vi "Geometrical Analysis with Linear Programming.vi"() -> ()   [LabVIEW 2023]
doc: "Determines the solution of a linear programming problem and displays the solution."
uses:
  <vilib>/gmath/NI_Gmath.lvlib
panel:
  in  "Subject to constraints":string[](array[string])=["-x1 -x2<=-.6", "-x1 -1.5*x2<=-.65", "-x1 -2*x2<=-.8", "-x1 -4*x2<=-1.2", "0.1*x1 +0.2*x2>=.01"]
  out "Solution (x1,x2)":dbl[](array[numeric]) format="%#.6g"
  in  "Optimization Problem":u16(ring) items=["Maximize", "Minimize"]
  in  "Objective Function":string="z= x1+1*x2"
  in  "Tab Control":enum32{"Table Notation", "Solution"}(tab)=enum."Solution"
  out "C":dbl[](array[numeric])
  out "B":dbl[](array[numeric])
  out "M":dbl[][](array[numeric])
  out "Linear Programming":cluster{"X":dbl[], "Y":dbl[]}[](graph)
  in  "Stop":bool
  out "Optimum Cost (z)":dbl=0.7600000076 format="%0.2f"
  # "Overview: Determines the solution of a linear programming problem of 2 variables and displays the solution graphically. \nRequirements: LabVIEW Full Development System\nInstructions: \n1. Run the VI and observe the graph on the Solution tab. Change the Objective function or Optimization Problem and verify the results.\n3. Click Stop to stop the VI."
  # "x1, x2 >= 0"
  # "x1"
  # "x2"
  # "The Linear Programming Equation Simplex Method VI requires you to obtain the equations in the format:\nc.x=max!;\nm.x>=b;\nx>=0."
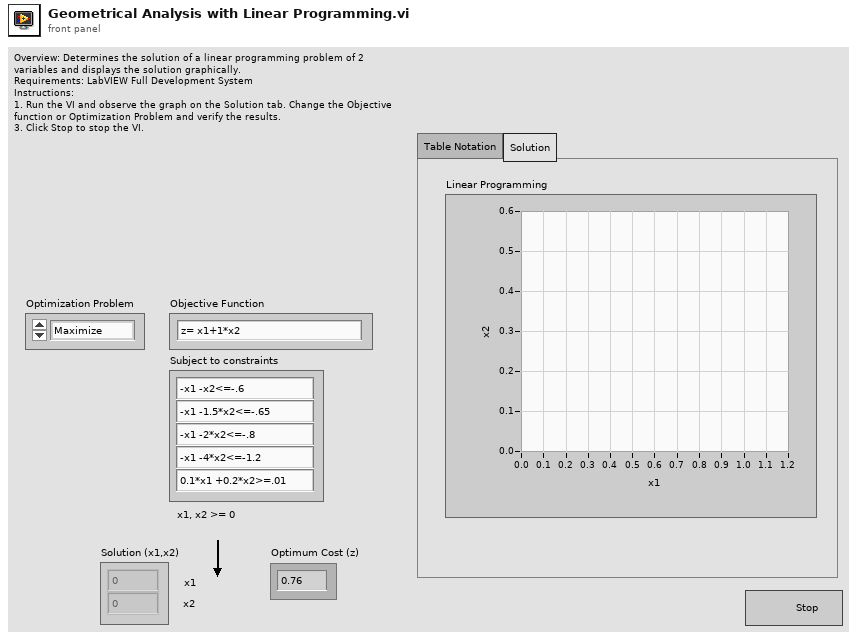
[diagram p1: front panel]
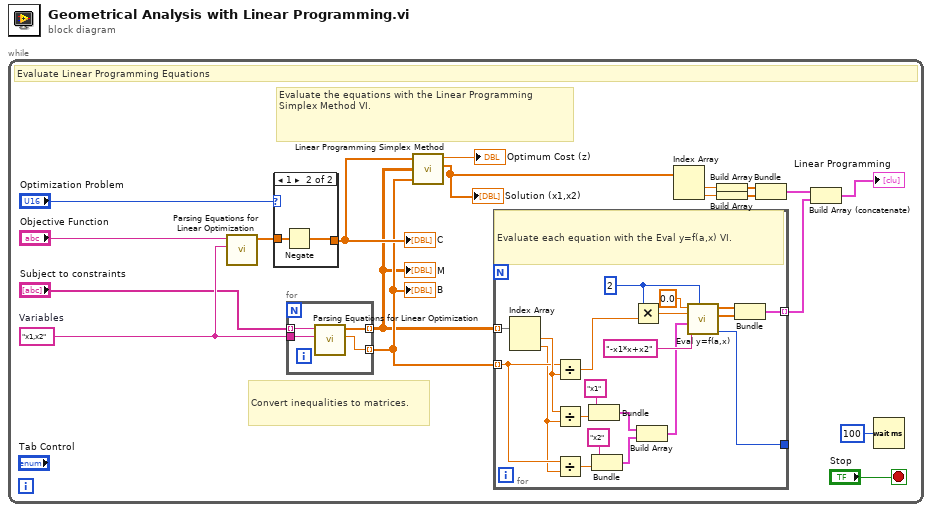
[diagram p0: block diagram]
diagram:
  n1 = while {
    stop <- "Stop" stop-if-true
    w16 = "x1,x2"  # Variables
    # "Convert inequalities to matrices."
    # "Evaluate the equations with the Linear Programming Simplex Method VI."
    # "Evaluate Linear Programming Equations"
    n2 = call "Parsing Equations for Linear Optimization.vi"("Variables"=w16, "Equation"="Objective Function") -> ("Vector"=w18:dbl[])  [unwired: 4 in, 5 out]
    n3 = case shown="1" "Optimization Problem" {
      tunnel: w18 -> [w44 w46]
      tunnel: [w44 w45] -> w17
      frame 0, Default {
      }
      frame 1 {
        n4 = Negate(x=w46) -> (-x=w45:dbl[])
      }
    }
    "C" <- w17
    n5 = for {
      tunnel: w16 -> [w23]
      tunnel: [w22] -> w4 mode=indexing
      tunnel: [w21] -> w15 mode=indexing
      tunnel: "Subject to constraints" -> [w20] mode=indexing
      # "Convert inequalities to matrices"
      n6 = call "Parsing Equations for Linear Optimization.vi"("Variables"=w23, "Equation"=w20) -> ("left side"=w21:dbl, "Vector"=w22:dbl[])  [unwired: 4 in, 4 out]
    }
    "B" <- w15
    "M" <- w4
    n7 = call <vilib>:"Linear Programming Simplex Method.vi"("C"=w17, "M"=w4, "B"=w15) -> ("maximum"=→"Optimum Cost (z)":dbl, "X"=w9:dbl[])  [unwired: 2 out]
    "Solution (x1,x2)" <- w9
    n8 = for {
      tunnel: w4 -> [w43] mode=indexing
      tunnel: w15 -> [w40] mode=indexing
      tunnel: [w34] -> w13 mode=indexing
      tunnel: [w27] -> _
      w24 = 2
      # "Evaluate each equation with the Eval y=f(a,x) VI."
      n9 = Index Array(array=w43) -> (element #1=w42:dbl, element #2=w29:dbl)  [unwired: 2 in]
      n10 = Divide(x=w40, y=w42) -> (x/y=w33:dbl)
      n11 = Divide(x=w42, y=w29) -> (x/y=w41:dbl)
      n12 = Divide(x=w40, y=w29) -> (x/y=w39:dbl)
      n13 = Bundle("x1", w41) -> (w38:cluster{string, dbl})  [unwired: 1 in]
      n14 = Bundle("x2", w39) -> (w37:cluster{string, dbl})  [unwired: 1 in]
      n15 = Multiply(x=w24, y=w33) -> (x*y=w32:dbl)
      n16 = Build Array(w38, w37) -> (w30:cluster{string, dbl}[])
      n17 = call <vilib>:"Eval y=f(a,x).vi"("number of points"=w24, "formula"="-x1*x+x2", "Parameters"=w30, "end"=w32, "start"=0.0) -> ("error"=w27:i32, "Y"=w35:dbl[], "X"=w36:dbl[])  [unwired: 1 out]
      n18 = Bundle("X"=w36, "Y"=w35) -> (w34:cluster{"X":dbl[], "Y":dbl[]})  [unwired: 1 in]
    }
    n19 = Index Array(array=w9) -> (element #1=w10:dbl, element #2=w6:dbl)  [unwired: 2 in]
    n20 = Build Array(w10) -> (w11:dbl[])
    n21 = Build Array(w6) -> (w12:dbl[])
    n22 = Bundle(w11, w12) -> (w14:cluster{dbl[], dbl[]})  [unwired: 1 in]
    n23 = Build Array (concatenate)(w14, w13) -> (→"Linear Programming":cluster{"X":dbl[], "Y":dbl[]}[])
    n24 = Wait (ms)(milliseconds to wait=u32 100) -> ()  [unwired: 1 out]
  }
